vi "gyroAvailable.vi"() -> (0 "x << y":i16)   [LabVIEW 2016]
uses:
  #defines.ctl
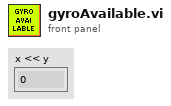
[diagram p1: front panel]
types:
  T1 = typedef "#defines.ctl" = i8
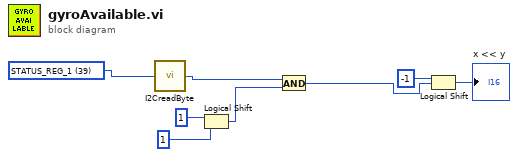
[diagram p0: block diagram]
diagram:
  w8 = T1 39 items=["CTRL_REG9"=35, "STATUS_REG_1"=39, "OUT_X_L_XL"=40, "FIFO_CTRL"=46, "FIFO_SRC"=47, "CTRL_REG4"=30, "OUT_X_L_G"=24, "OUT_TEMP_L"=21, "INT_GEN_SRC_G"=20, "ORIENT_CFG_G"=19, "CTRL_REG3_G"=18, "CTRL_REG2_G"=17, "CTRL_REG1_G"=16, "WHO_AM_I_XG"=15] ("Ring")
  n1 = call "I2CreadByte.vi"("subAddress"=w8) -> ("data"=w7:u8)
  n2 = Logical Shift(y=i16 1, x=i16 1) -> (x << y=w4:i16)
  n3 = And(x=w7, y=w4) -> (x .and. y?=w2:i16)
  n4 = Logical Shift(y=i16 -1, x=w2) -> (x << y=→"x << y":i16)
